vi "Workshop Exercise 1 Solution.vi"() -> ()   [LabVIEW 2019]
doc: "ss"
panel:
  out "Less than or Equal to Zero":dbl[](array[numeric])
  out "Greater than Zero":dbl[](array[numeric])
  in  "Input Array":dbl[](array[numeric])=[156.23, -11.0, -9.2, 0.0, 3.01, -2.0, 0.0, 35.62]
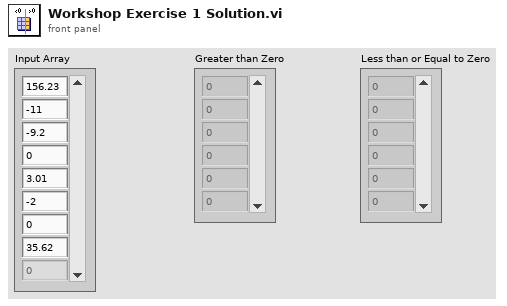
[diagram p1: front panel]
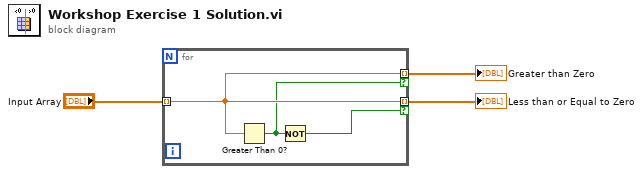
[diagram p0: block diagram]
diagram:
  n1 = for {
    tunnel: "Input Array" -> [w6] mode=indexing
    tunnel: [w6] -> w2 mode=indexing if=w5
    tunnel: [w6] -> w1 mode=indexing if=w4
    n2 = Greater Than 0?(x=w6) -> (x > 0?=w5:bool)
    n3 = Not(x=w5) -> (.not. x?=w4:bool)
  }
  "Greater than Zero" <- w2
  "Less than or Equal to Zero" <- w1
